vi "Keep good hits.vi"(8 "Collection in":T2(array[cluster]), 11 "Array":T1[](array[typedef])) -> (0 "Collection out":T2(array[cluster]))   [LabVIEW 2016]
uses:
  Typedefs/Coincidence.ctl
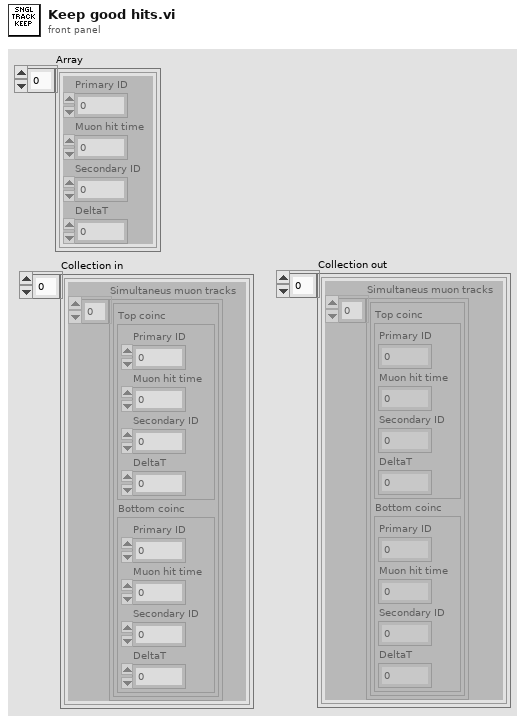
[diagram p1: front panel]
types:
  T1 = typedef "Coincidence.ctl" = cluster{"Primary ID":i8, "Muon hit time":u64, "Secondary ID":i8, "DeltaT":i32}
  T2 = cluster{"Simultaneus muon tracks":cluster{"Top coinc":T1, "Bottom coinc":T1}[]}[]
  T3 = cluster{"Simultaneus muon tracks":cluster{"Top coinc":T1, "Bottom coinc":T1}[]}
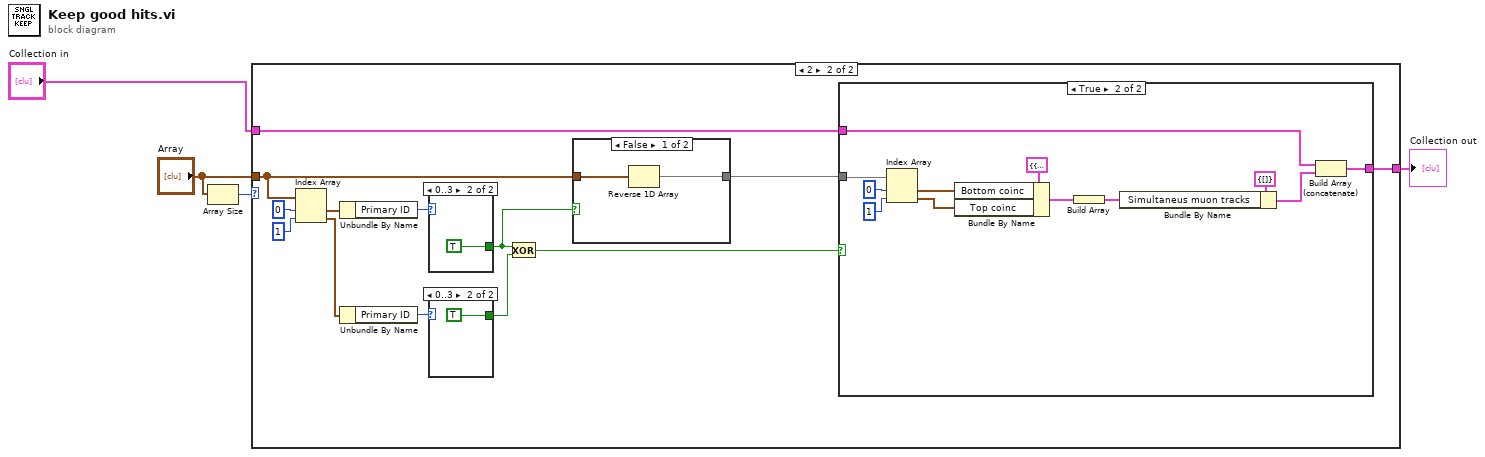
[diagram p0: block diagram]
diagram:
  n1 = Array Size(array="Array") -> (size(s)=w3:i32)
  n2 = case shown="2" w3 {
    tunnel: "Array" -> [_ w7]
    tunnel: "Collection in" -> [w5 w11]
    tunnel: [w5 w9] -> w1
    frame Default {
    }
    frame 2 {
      n3 = Index Array(array=w7, index #1=0 ("index"), index #2=1 ("index")) -> (element #1=w16:T1, element #2=w15:T1)
      n4 = Unbundle By Name(w16) -> ("Primary ID"=w14:i8)
      n5 = Unbundle By Name(w15) -> ("Primary ID"=w13:i8)
      n6 = case shown="0..3" w14 {
        tunnel: [_ TRUE] -> w8
        frame Default {
        }
        frame 0..3 {
        }
      }
      n7 = case shown="0..3" w13 {
        tunnel: [_ TRUE] -> w12
        frame Default {
        }
        frame 0..3 {
        }
      }
      n8 = Exclusive Or(1:w12, 2:w8) -> (0:w10:bool)
      n9 = case shown="False" w8 {
        tunnel: w7 -> [w20 w21]
        tunnel: [w19 w21] -> w6
        frame False {
          n10 = Reverse 1D Array(array=w20) -> (reversed array=w19:T1[])
        }
        frame True {
        }
      }
      n11 = case shown="True" w10 {
        tunnel: w11 -> [w22 w34]
        tunnel: w6 -> [_ w28]
        tunnel: [w22 w33] -> w9
        frame False {
        }
        frame True {
          n12 = Index Array(array=w28, index #1=0 ("index"), index #2=1 ("index")) -> (element #1=w27:T1, element #2=w26:T1)
          n13 = Bundle By Name(cluster=cluster{"Top coinc":T1, "Bottom coinc":T1} {"Top coinc"={"Primary ID"=0, "Muon hit time"=0, "Secondary ID"=0, "DeltaT"=0}, "Bottom coinc"={"Primary ID"=0, "Muon hit time"=0, "Secondary ID"=0, "DeltaT"=0}} ("Muon event"), "Bottom coinc"=w27, "Top coinc"=w26) -> (w25:cluster{"Top coinc":T1, "Bottom coinc":T1})
          n14 = Build Array(w25) -> (w24:cluster{"Top coinc":T1, "Bottom coinc":T1}[])
          n15 = Bundle By Name(cluster=T3 {"Simultaneus muon tracks"=[]} ("Simultaneus muon tracks"), "Simultaneus muon tracks"=w24) -> (w23:T3)
          n16 = Build Array (concatenate)(w34, w23) -> (w33:T2)
        }
      }
    }
  }
  "Collection out" <- w1
